vi "Init(Camera).vi"(8 "error in (no error)":errorcluster, 10 "Camera_Settings_Ref":refnum<vi>, 11 "Session in":T1) -> (0 "error out":errorcluster, 3 "Session out":T1)   [LabVIEW 2020]
uses:
  <vilib>/userDefined/High Color/IMAQdx.ctl
  Controls/Camera_Settings.ctl
  <resource>/objmgr/imaqdx.rc
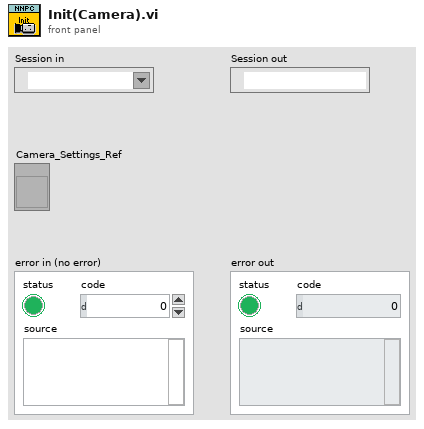
[diagram p1: front panel]
types:
  T1 = typedef "IMAQdx.ctl" = refnum<k21>
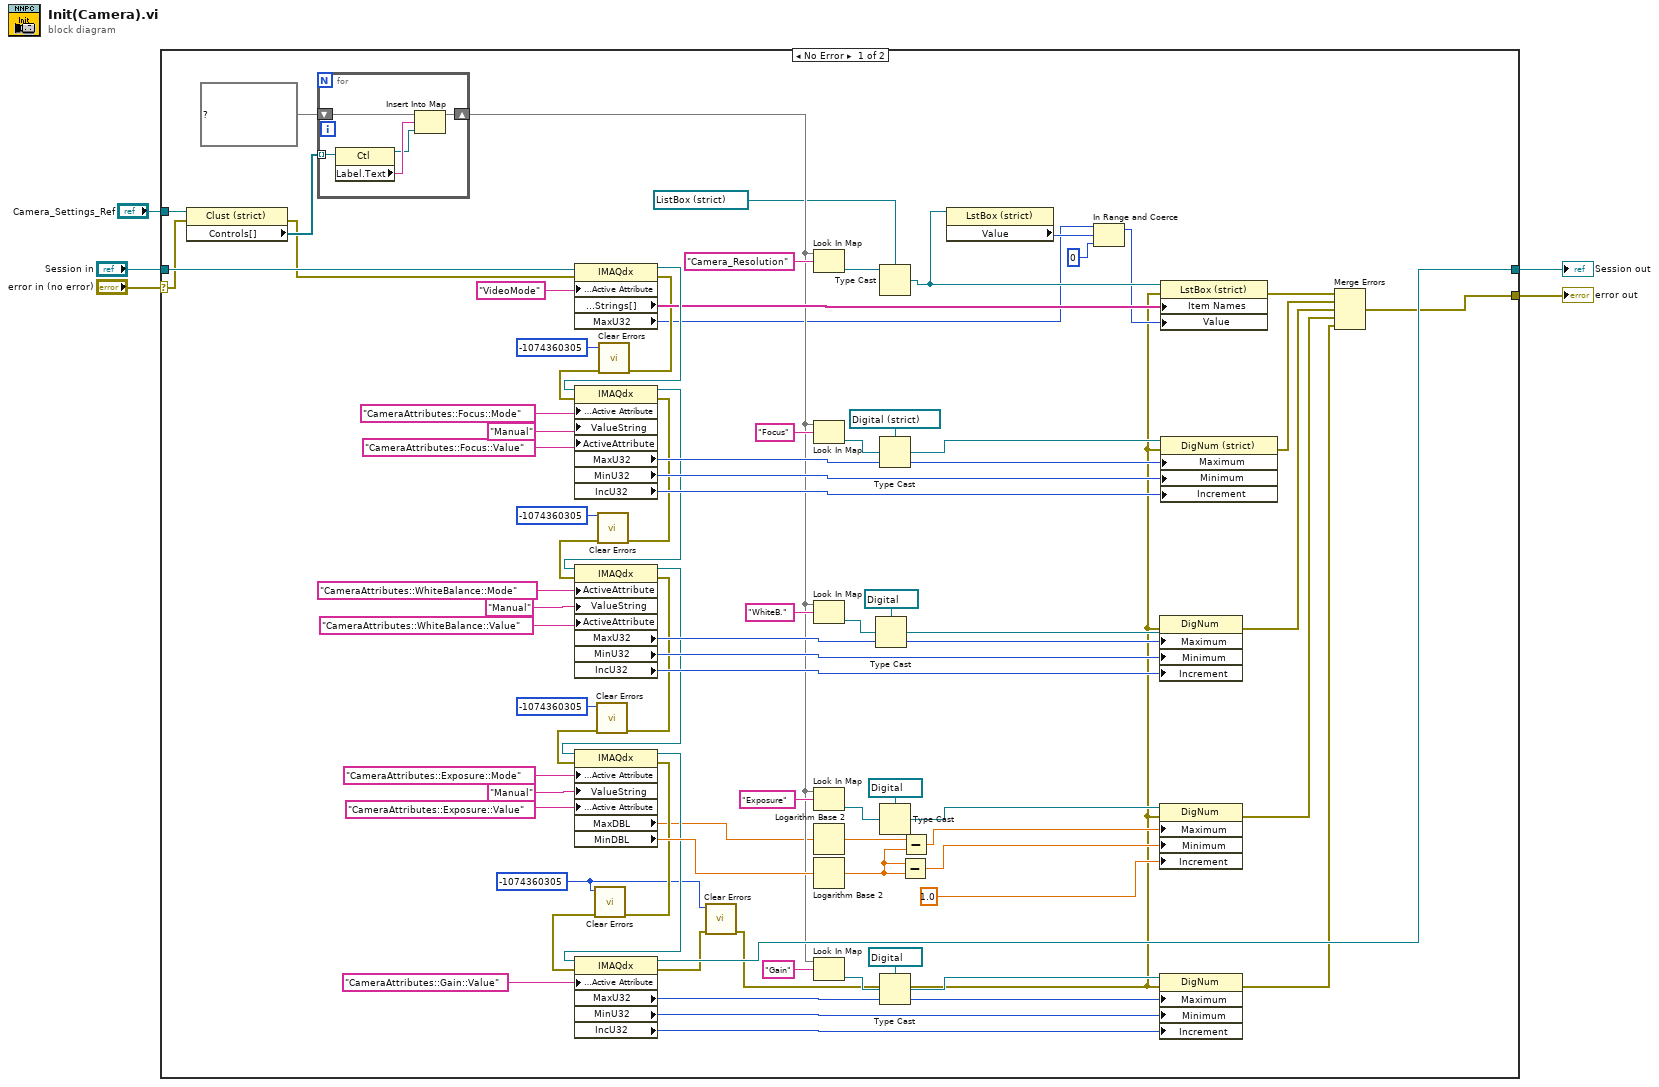
[diagram p0: block diagram]
diagram:
  n1 = case shown="No Error" "error in (no error)" {
    selector: "error in (no error)" -> [w47 w96]
    tunnel: [w78 w95] -> w5
    tunnel: [w25 w96] -> w4
    tunnel: "Camera_Settings_Ref" -> [w69 _]
    tunnel: "Session in" -> [w48 w95]
    frame No Error {
      w6 = -1074360305 ("specific error code to clear (0: all)")
      n2 = property class="Clust (strict)"(reference=w69, error in=w47) -> (error out=w46:errorcluster, "Controls[]"=w68:refnum<vi>[])  [unwired: 1 out]
      n3 = for {
        tunnel: w68 -> [w94] mode=indexing
        shift-right: [w90] -> w35
        shift-left: map{string, refnum<vi>} {} ("map") -> [w93]
        n4 = property class="Ctl"(reference=w94) -> (reference out=w91:refnum<vi>, "Label.Text"=w92:string)  [unwired: 1 in, 1 out]
        n5 = Insert Into Map(map in=w93, key=w92, value=w91) -> (map out=w90:map{string, refnum<vi>})  [unwired: 2 out]
      }
      n6 = property class="IMAQdx"(reference=w48, error in=w46, "Camera Attributes:Active Attribute"="VideoMode" ("ActiveAttribute")) -> (reference out=w72:T1, error out=w33:errorcluster, "Camera Attributes:Enum:Strings[]"=w71:string[], "MaxU32"=w10:u32)
      n7 = call <vilib>:"Clear Errors.vi"("error in (no error)"=w33, "specific error code to clear (0: all)"=-1074360305) -> ("error out"=w24:errorcluster)  [unwired: 4 in, 1 out]
      n8 = property class="IMAQdx"(reference=w72, error in=w24, "Camera Attributes:Active Attribute"="CameraAttributes::Focus::Mode" ("ActiveAttribute"), "ValueString"="Manual", "ActiveAttribute"="CameraAttributes::Focus::Value") -> (reference out=w54:T1, error out=w34:errorcluster, "MaxU32"=w87:u32, "MinU32"=w88:u32, "IncU32"=w89:u32)
      n9 = call <vilib>:"Clear Errors.vi"("error in (no error)"=w34, "specific error code to clear (0: all)"=-1074360305) -> ("error out"=w23:errorcluster)  [unwired: 4 in, 1 out]
      n10 = property class="IMAQdx"(reference=w54, error in=w23, "ActiveAttribute"="CameraAttributes::WhiteBalance::Mode", "ValueString"="Manual", "ActiveAttribute"="CameraAttributes::WhiteBalance::Value") -> (reference out=w53:T1, error out=w32:errorcluster, "MaxU32"=w58:u32, "MinU32"=w59:u32, "IncU32"=w60:u32)
      n11 = call <vilib>:"Clear Errors.vi"("error in (no error)"=w32, "specific error code to clear (0: all)"=-1074360305) -> ("error out"=w22:errorcluster)  [unwired: 4 in, 1 out]
      n12 = property class="IMAQdx"(reference=w53, error in=w22, "Camera Attributes:Active Attribute"="CameraAttributes::Exposure::Mode" ("ActiveAttribute"), "ValueString"="Manual", "Camera Attributes:Active Attribute"="CameraAttributes::Exposure::Value" ("ActiveAttribute")) -> (reference out=w77:T1, error out=w31:errorcluster, "MaxDBL"=w17:dbl, "MinDBL"=w83:dbl)
      n13 = call <vilib>:"Clear Errors.vi"("error in (no error)"=w31, "specific error code to clear (0: all)"=w6) -> ("error out"=w21:errorcluster)  [unwired: 4 in, 1 out]
      n14 = property class="IMAQdx"(reference=w77, error in=w21, "Camera Attributes:Active Attribute"="CameraAttributes::Gain::Value" ("ActiveAttribute")) -> (reference out=w78:T1, error out=w8:errorcluster, "MaxU32"=w76:u32, "MinU32"=w75:u32, "IncU32"=w74:u32)
      n15 = call <vilib>:"Clear Errors.vi"("error in (no error)"=w8, "specific error code to clear (0: all)"=w6) -> ("error out"=w7:errorcluster)  [unwired: 4 in, 1 out]
      n16 = Look In Map(map=w35, key="Camera_Resolution") -> (value=w15:refnum<vi>)  [unwired: 1 in, 1 out]
      n17 = Look In Map(map=w35, key="Focus") -> (value=w39:refnum<vi>)  [unwired: 1 in, 1 out]
      n18 = Look In Map(map=w35, key="WhiteB.") -> (value=w38:refnum<vi>)  [unwired: 1 in, 1 out]
      n19 = Look In Map(map=w35, key="Exposure") -> (value=w37:refnum<vi>)  [unwired: 1 in, 1 out]
      n20 = Logarithm Base 2(1:w17) -> (0:w81:dbl)
      n21 = Logarithm Base 2(1:w83) -> (0:w82:dbl)
      n22 = Look In Map(map=w35, key="Gain") -> (value=w36:refnum<vi>)  [unwired: 1 in, 1 out]
      n23 = Type Cast(type=refnum<vi> refnum ("DigNum Refnum"), x=w38) -> (*(type *) &x=w62:refnum<vi>)
      n24 = Type Cast(type=refnum<vi> refnum ("Camera_Resolution"), x=w15) -> (*(type *) &x=w13:refnum<vi>)
      n25 = Type Cast(type=refnum<vi> refnum ("DigNum Refnum 5"), x=w39) -> (*(type *) &x=w61:refnum<vi>)
      n26 = Type Cast(type=refnum<vi> refnum ("DigNum Refnum"), x=w37) -> (*(type *) &x=w64:refnum<vi>)
      n27 = Type Cast(type=refnum<vi> refnum ("DigNum Refnum"), x=w36) -> (*(type *) &x=w63:refnum<vi>)
      n28 = Subtract(x=w82, y=w82) -> (x-y=w85:dbl)
      n29 = Subtract(x=w81, y=w82) -> (x-y=w84:dbl)
      n30 = property on="Property Node" class="LstBox (strict)"(reference=w13) -> ("Value"=w11:i32)  [unwired: 1 in, 2 out]
      n31 = In Range and Coerce(upper limit=w10, x=w11, lower limit=u32 0) -> (coerced(x)=w12:u32)  [unwired: 1 out]
      n32 = property on="Property Node" class="DigNum"(reference=w62, error in=w7, "Maximum"=w58, "Minimum"=w59, "Increment"=w60) -> (error out=w28:errorcluster)  [unwired: 1 out]
      n33 = property on="Property Node" class="DigNum"(reference=w64, error in=w7, "Maximum"=w84, "Minimum"=w85, "Increment"=1.0 ("Data Entry Limits:Increment")) -> (error out=w27:errorcluster)  [unwired: 1 out]
      n34 = property on="Property Node" class="DigNum"(reference=w63, error in=w7, "Maximum"=w76, "Minimum"=w75, "Increment"=w74) -> (error out=w26:errorcluster)  [unwired: 1 out]
      n35 = property on="Property Node" class="LstBox (strict)"(reference=w13, error in=w7, "Item Names"=w71, "Value"=w12) -> (error out=w30:errorcluster)  [unwired: 1 out]
      n36 = property on="Property Node" class="DigNum (strict)"(reference=w61, error in=w7, "Maximum"=w87, "Minimum"=w88, "Increment"=w89) -> (error out=w29:errorcluster)  [unwired: 1 out]
      n37 = Merge Errors(w30, w29, w28, w27, w26) -> (w25:errorcluster)
    }
    frame Error {
    }
  }
  "Session out" <- w5
  "error out" <- w4
